vi "Data_SetType.vi"(8 "error in":errorcluster, 10 "type":T1=enum."File", 11 "data":variant) -> (0 "error out":errorcluster, 3 "data out":variant)   [LabVIEW 2017, in "FileManager.lvlib"]
uses:
  <vilib>/addons/InsightCM/Devices/Shared/Common/FileManager/FileManager.lvlib
  <vilib>/addons/InsightCM/Devices/Shared/Common/FileManager/controls/DataType.ctl
  <vilib>/addons/InsightCM/Devices/Shared/Common/FileManager/controls/DataPropertyNames.ctl
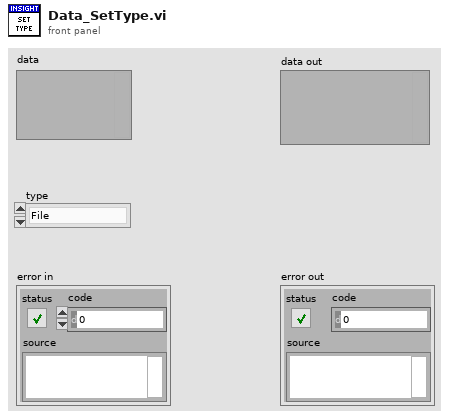
[diagram p1: front panel]
types:
  T1 = typedef "FileManager.lvlib/DataType.ctl" = enum16{"Default", "File", "InMemory", "EventRef", "EventRefFile"}
  T2 = typedef "DataPropertyNames.ctl" = enum16{"Type", "EventRef", "FilePath", "DataGroup", "AcquisitionTimestamp", "StreamId", "StreamBlock", "TrendPointsOnly", "ExtraLargeFile"}
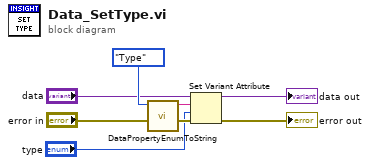
[diagram p0: block diagram]
diagram:
  n1 = call <vilib>:"DataPropertyEnumToString.vi"("property"=DataPropertyNames."Type" ("Names")) -> ("string"=w5:string)  [unwired: 10 in]
  n2 = Set Variant Attribute(Variant="data", name=w5, value="type", error in="error in") -> (Variant out=→"data out":variant, error out=→"error out":errorcluster)  [unwired: 1 out]
